vi "Properties Consolidate_As In Node.vi"(7 "Action":T1, 8 "Class":string, 11 "Property Info Array":T3(array[cluster])) -> (3 "Property Info Out":T2(array[cluster]))   [LabVIEW 2023]
uses:
  controls/action enum.ctl
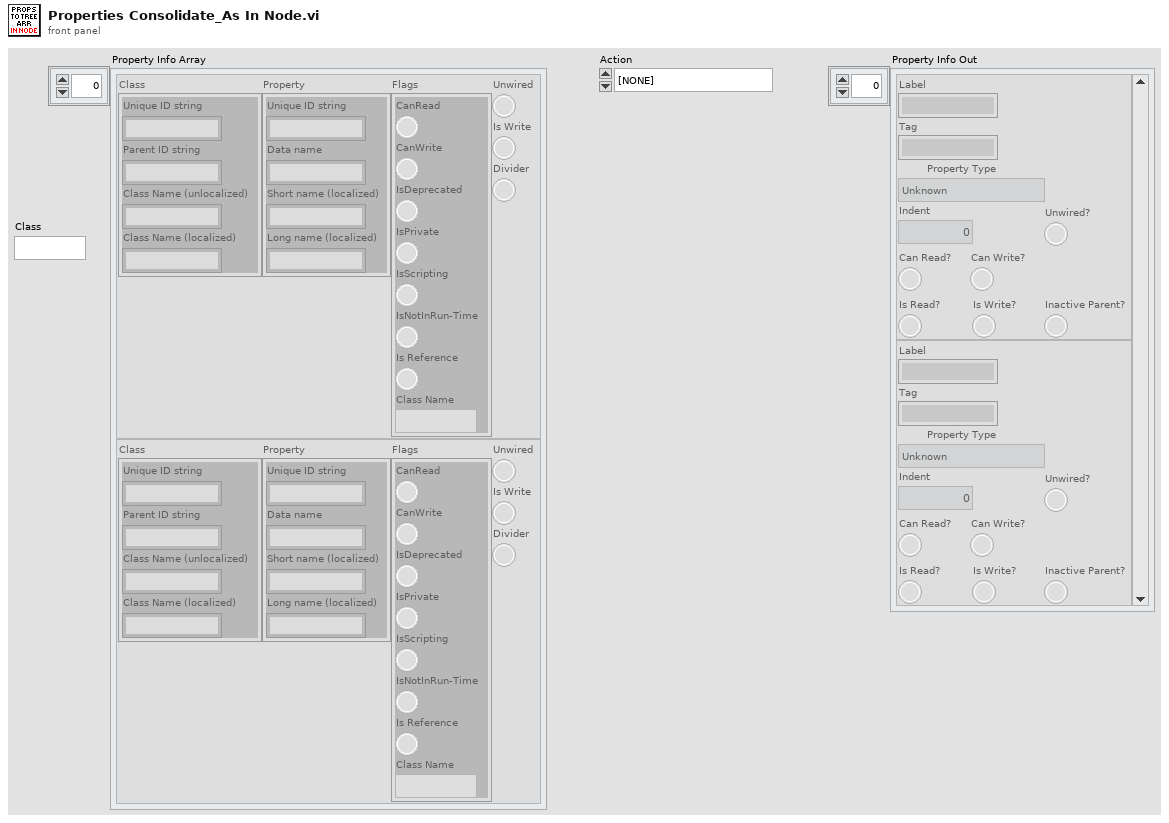
[diagram p1: front panel]
types:
  T1 = typedef "action enum.ctl" = enum16{"[NONE]", "Wire Bundle", "Wire Unbundle", "Terminal Unbundle", "Terminal Bundle", "Bundler Move Up", "Bundler Move Down", "Bundler Insert", "Bundler Remove", "Bundler Remove Unwired", "Bundler Rearrange", "In Place Insert", "In Place Remove", "In Place Remove Unwired", "In Place Rearrange", "Wire Properties", "Wire Method", "Terminal Properties", "Terminal Method", "Property Move Up", "Property Move Down", "Properties Insert", "Properties Remove", "Properties Remove Unwired", "Properties Rearrange", "Method Change", "Class for Constant", "Class For Control", "Class For Node", "Class Name to Clipboard"}
  T2 = cluster{"Label":string, "Tag":string, "Property Type":enum16{"Unknown", "Base", "Scripting", "Private", "Deprecated", "None", "Divider"}, "Indent":u16, "Can Read?":bool, "Can Write?":bool, "Is Read?":bool, "Is Write?":bool, "Inactive Parent?":bool, "Unwired?":bool}[]
  T3 = cluster{"Class":cluster{"Unique ID string":string, "Parent ID string":string, "Class Name (unlocalized)":string, "Class Name (localized)":string}, "Property":cluster{"Unique ID string":string, "Data name":string, "Short name (localized)":string, "Long name (localized)":string}, "Flags":cluster{"CanRead":bool, "CanWrite":bool, "IsDeprecated":bool, "IsPrivate":bool, "IsScripting":bool, "IsNotInRun-Time":bool, "Is Reference":bool, "Class Name":string}, "Divider":bool, "Is Write":bool, "Unwired":bool}[]
  T4 = cluster{"Label":string, "Tag":string, "Property Type":enum16{"Unknown", "Base", "Scripting", "Private", "Deprecated", "None", "Divider"}, "Indent":u16, "Can Read?":bool, "Can Write?":bool, "Is Read?":bool, "Is Write?":bool, "Inactive Parent?":bool, "Unwired?":bool}
  T5 = cluster{"Unique ID string":string, "Data name":string, "Short name (localized)":string, "Long name (localized)":string}
  T6 = enum16{"Unknown", "Base", "Scripting", "Private", "Deprecated", "None", "Divider"}
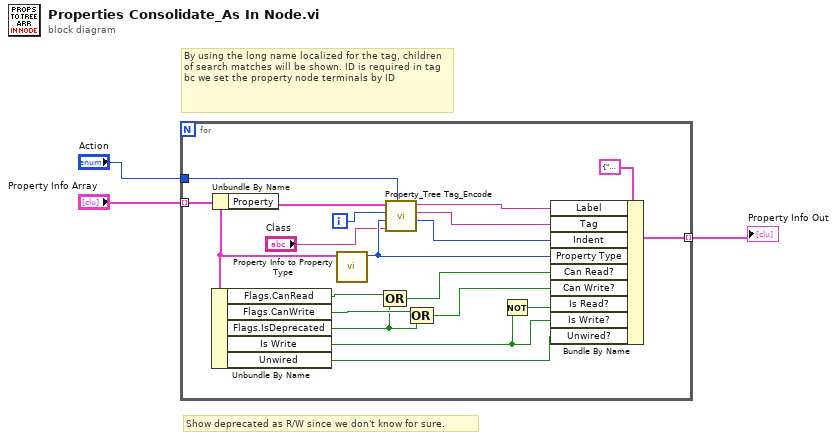
[diagram p0: block diagram]
diagram:
  # "Show deprecated as R/W since we don't know for sure."
  # "By using the long name localized for the tag, children of search matches will be shown. ID is required in tag bc we set the property node terminals by ID"
  n1 = for {
    tunnel: "Property Info Array" -> [w16] mode=indexing
    tunnel: [w14] -> w1 mode=indexing
    tunnel: "Action" -> [w20]
    i -> [w19]
    n2 = Unbundle By Name(w16) -> ("Flags.CanRead"=w8:bool, "Flags.CanWrite"=w6:bool, "Flags.IsDeprecated"=w5:bool, "Is Write"=w10:bool, "Unwired"=w9:bool)
    n3 = Unbundle By Name(w16) -> ("Property"=w22:T5)
    n4 = call "Property Info to Property Type.vi"("Cluster"=w16) -> ("Property Type"=w18:T6)  [unwired: 10 in]
    n5 = Compound Arithmetic op=OR(w8, w5) -> (w7:bool)
    n6 = call "Property_Tree Tag_Encode.vi"("Action"=w20, "Class"="Class", "Property Type"=w18, "Index"=w19, "Method/Property Info"=w22) -> ("Indent"=w21:i32, "Tag"=w15:string, "Bare name"=w17:string)  [unwired: 2 in, 2 out]
    n7 = Compound Arithmetic op=OR(w6, w5) -> (w4:bool)
    n8 = Not(x=w10) -> (.not. x?=w11:bool)
    n9 = Bundle By Name(cluster=T4 {"Label"="", "Tag"="", "Property Type"=enum."Unknown", "Indent"=0, "Can Read?"=FALSE, "Can Write?"=FALSE, "Is Read?"=FALSE, "Is Write?"=FALSE, "Inactive Parent?"=FALSE, "Unwired?"=FALSE} ("Cluster 3"), "Label"=w17, "Tag"=w15, "Indent"=w21, "Property Type"=w18, "Can Read?"=w7, "Can Write?"=w4, "Is Read?"=w11, "Is Write?"=w10, "Unwired?"=w9) -> (w14:T4)
  }
  "Property Info Out" <- w1
